vi "RPC Method TestService Method2.vi"(8 "error in (no error)":errorcluster, 11 "OOP Server in":refnum<class "TestService.lvclass">) -> (0 "error out":errorcluster, 3 "OOP Server out":refnum<class "TestService.lvclass">)   [LabVIEW 2021, in "test_service_server.lvlib" / "TestService.lvclass"]
uses:
  TestService.lvclass
  test_service_server.lvlib
  RPC Messages/test_service_Method2Response.ctl
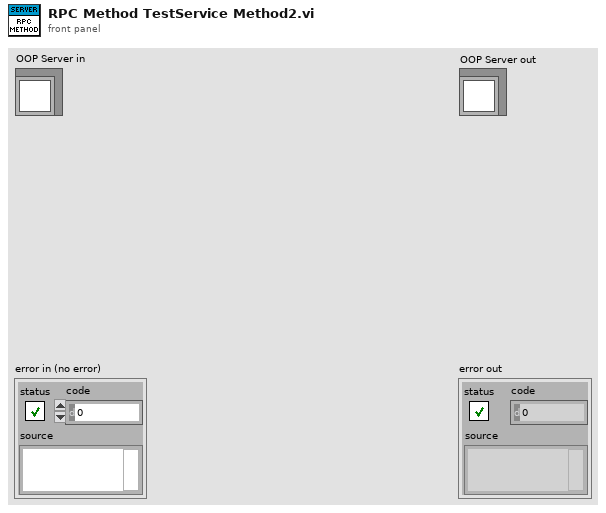
[diagram p1: front panel]
types:
  T1 = typedef "test_service_server.lvlib/test_service_Method2Response.ctl" = cluster{"timestamp_request":u64, "timestamp":u64}
  T2 = typedef "test_service_server.lvlib/TestService.lvclass/Server Internal UEs.ctl" = cluster{"TestService Method1 Internal UE":refnum<user-event>, "TestService Method2 Internal UE":refnum<user-event>, "TestService Method3 Internal UE":refnum<user-event>, "TestService Method4 Internal UE":refnum<user-event>}
  T3 = typedef "test_service_server.lvlib/TestService.lvclass/Server gRPC UEs.ctl" = cluster{"TestService Method1 gRPC UE":refnum<user-event>, "TestService Method2 gRPC UE":refnum<user-event>, "TestService Method3 gRPC UE":refnum<user-event>, "TestService Method4 gRPC UE":refnum<user-event>}
  T4 = typedef "grpc-lvsupport-release.lvlib/grpcId.ctl" = u64
  T5 = typedef "test_service_server.lvlib/test_service_Method2Request.ctl" = cluster{"timestamp":u64}
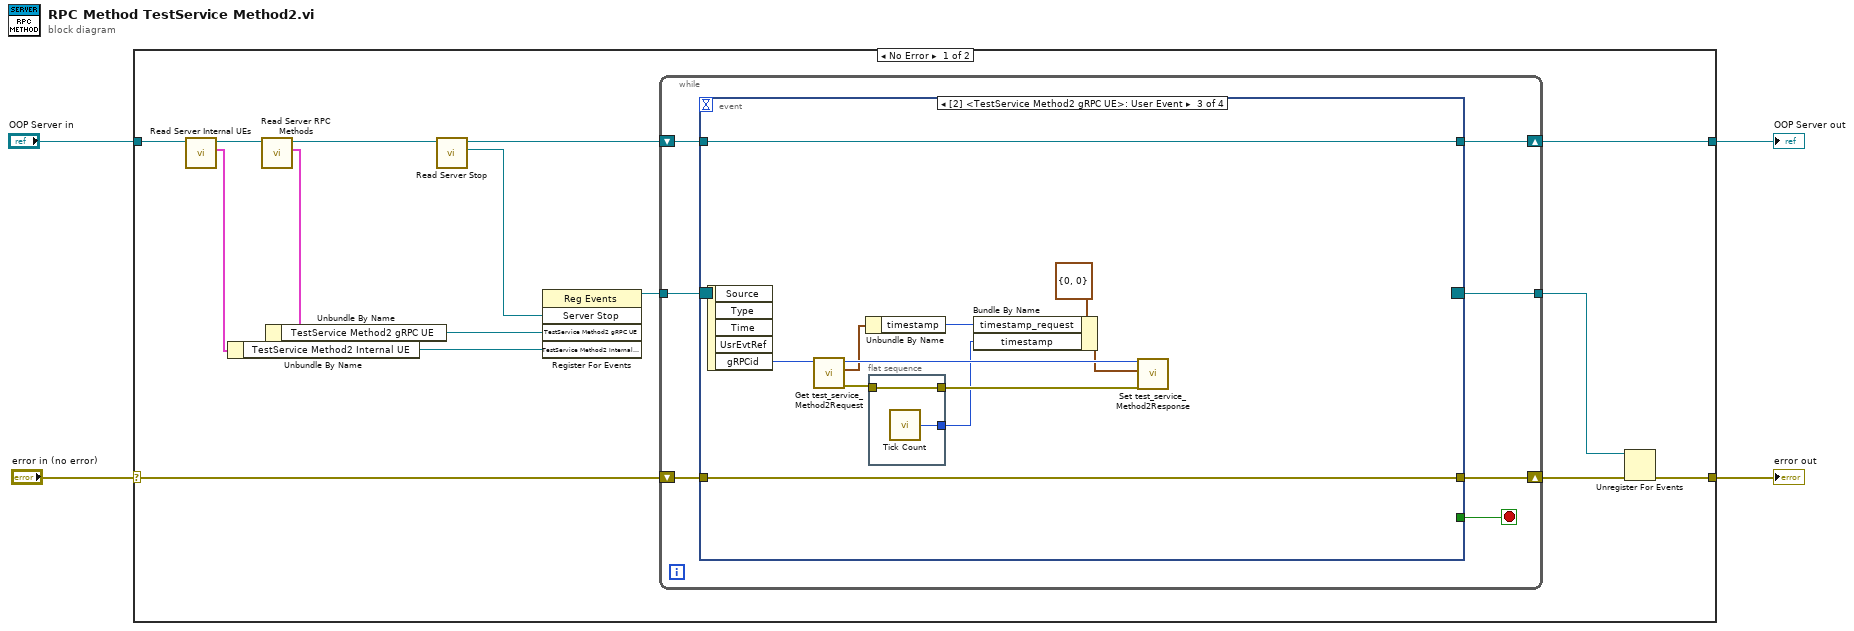
[diagram p0: block diagram]
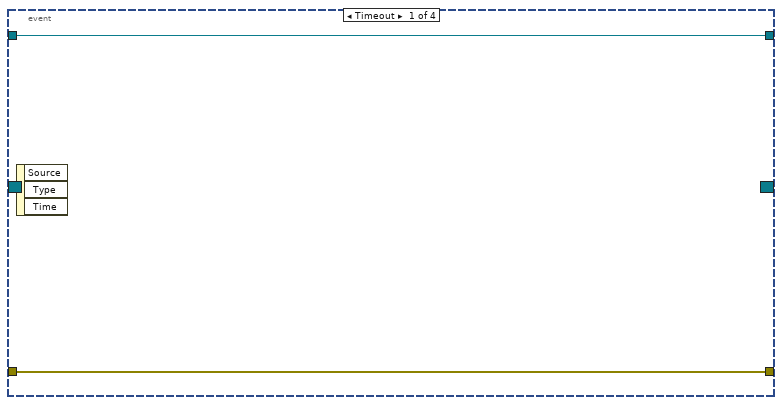
[diagram p2: hidden frame]
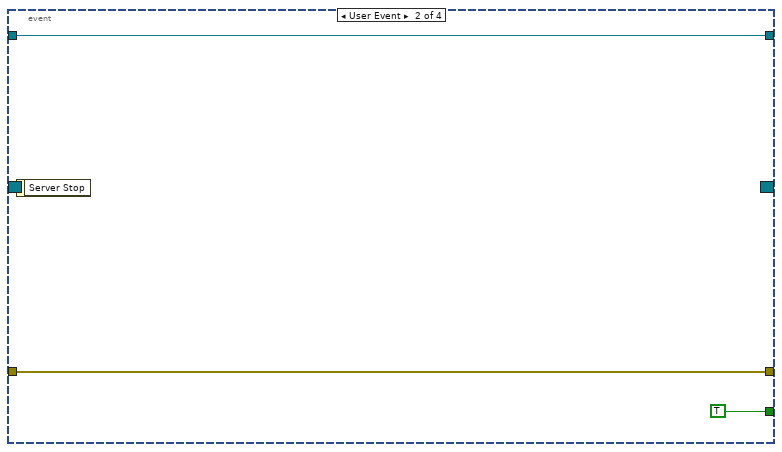
[diagram p3: hidden frame]
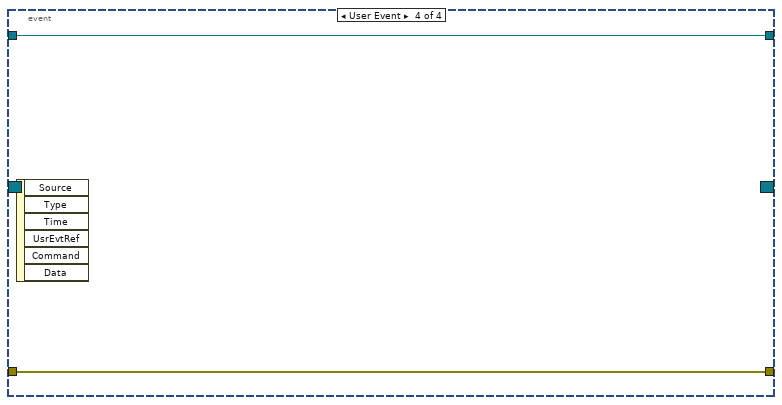
[diagram p4: hidden frame]
diagram:
  n1 = case shown="No Error" "error in (no error)" {
    selector: "error in (no error)" -> [w15 w48]
    tunnel: [w13 w48] -> w3
    tunnel: "OOP Server in" -> [w17 w47]
    tunnel: [w5 w47] -> w1
    frame No Error {
      n2 = call "Read Server Internal UEs.vi"("SignalGeneratorService in"=w17) -> ("Server Internal UEs"=w9:T2, "SignalGeneratorService out"=w16:refnum<class "TestService.lvclass">)  [unwired: 8 in, 1 out]
      n3 = Unbundle By Name ("Unbundle Internal UE")(w9) -> ("TestService Method2 Internal UE"=w8:refnum<user-event>)
      n4 = call "Read Server RPC Methods.vi"("SignalGeneratorService in"=w16) -> ("Server RPC Methods"=w11:T3, "SignalGeneratorService out"=w6:refnum<class "TestService.lvclass">)  [unwired: 8 in, 1 out]
      n5 = Unbundle By Name ("Unbundle gRPC UE")(w11) -> ("TestService Method2 gRPC UE"=w10:refnum<user-event>)
      n6 = call-dynamic "Read Server Stop.vi"("iService in"=w6) -> ("Server Stop"=w19:refnum<user-event>, "iService out"=w7:refnum<class "TestService.lvclass">)  [unwired: 8 in, 1 out]
      n7 = register-events(w19, w10, w8) -> (reference out=w18:refnum<event-registration>)  [unwired: 2 in, 1 out]
      n8 = while {
        tunnel: w18 -> [w26]
        tunnel: [w22] -> w12
        shift-right: [w23] -> w14
        shift-left: w15 -> [w24]
        shift-right: [w20] -> w5
        shift-left: w7 -> [w21]
        stop <- w25 stop-if-true
        n9 = event "RPC Method Event Structure" shown="[2] <TestService Method2 gRPC UE>: User Event" {
          selector: w26 -> [_ _ _ _]
          dyn-events: [_ _ _ _] -> w22
          timeout: _ -> [_ _ _ _]
          tunnel: [_ TRUE _ _] -> w25
          tunnel: w24 -> [w28 w30 w42 w46]
          tunnel: [w28 w30 w42 w46] -> w23
          tunnel: w21 -> [w27 w29 w41 w45]
          tunnel: [w27 w29 w41 w45] -> w20
          event Timeout {
            n10 = event-data() -> ()  [unwired: 1 in, 3 out]
          }
          event User Event {
            n11 = event-data() -> ()  [unwired: 1 in, 1 out]
          }
          event User Event {
            n12 = event-data() -> ("gRPCid"=w32:T4)  [unwired: 1 in, 4 out]
            n13 = call "Get test_service_Method2Request.vi"("gRPCid"=w32) -> ("error out"=w35:errorcluster, "package_templatemessage"=w39:T5, "gRPCid out"=w40:T4)  [unwired: 8 in]
            n14 = Unbundle By Name(w39) -> ("timestamp"=w37:u64)
            n15 = flat-sequence {
              tunnel: [w44] -> w34
              tunnel: w35 -> [w44]
              tunnel: [w43] -> w33
              frame #0 {
                n16 = call "Tick Count"() -> ("Tick Count(uSec)"=w43:u32)
              }
            }
            n17 = Bundle By Name(cluster=T1 {"timestamp_request"=0, "timestamp"=0} ("package_templatemessage"), "timestamp_request"=w37, "timestamp"=w33) -> (w36:T1)
            n18 = call "Set test_service_Method2Response.vi"("error in (no error)"=w34, "package_templatemessage"=w36, "gRPCid"=w40) -> ()  [unwired: 8 in, 1 out]
          }
          event User Event {
            n19 = event-data() -> ()  [unwired: 1 in, 6 out]
          }
        }
      }
      n20 = Unregister For Events(event registration refnum=w12, error in=w14) -> (error out=w13:errorcluster)
    }
    frame Error {
    }
  }
  "error out" <- w3
  "OOP Server out" <- w1
